vi "lugre.vi"(0 "stribeck velocity":dbl, 1 "bristle stiffness":dbl, 2 "bristle damping":dbl, 3 "viscous friction":dbl, 4 "stiction friction":dbl, 5 "columb friction":dbl, 6 "velocity":dbl, 8 "F before compensation":dbl, 9 "time sampling":dbl, 11 "tracking error":dbl, 13 "observer gain":dbl) -> (14 "F":dbl, 15 "compensated F":dbl)   [LabVIEW 2012]
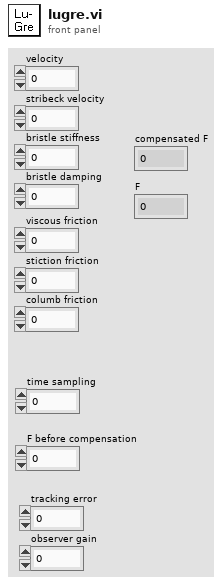
[diagram p1: front panel]
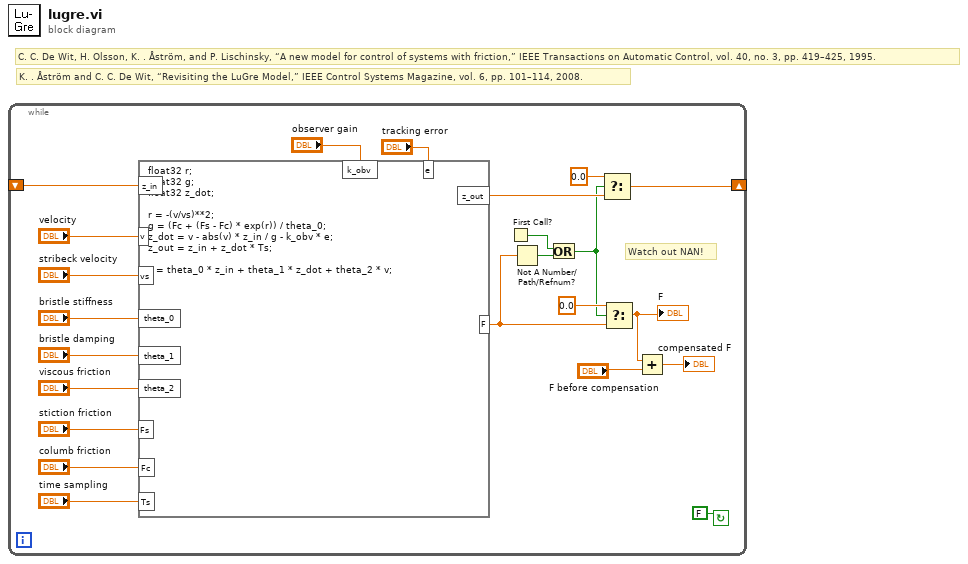
[diagram p0: block diagram]
diagram:
  # "K. . Åström and C. C. De Wit, “Revisiting the LuGre Model,” IEEE Control Systems Magazine, vol. 6, pp. 101–114, 2008."
  # "C. C. De Wit, H. Olsson, K. . Åström, and P. Lischinsky, “A new model for control of systems with friction,” IEEE Transactions on Automatic Control, vol. 40, no. 3, pp. 419–425, 1995."
  n1 = while {
    shift-right: [w4] -> _
    shift-left: _ -> [w14]
    stop <- FALSE continue-if-true
    # "Watch out NAN!"
    n2 = formula code="float32 r;\nfloat32 g;\nfloat32 z_dot;\n\nr = -(v/vs)**2;\ng = (Fc + (Fs - Fc) * exp(r)) / theta_0;\nz_dot = v - abs(v) * z_in / g - k_obv * e;\nz_out = z_in + z_dot * Ts;\n\nF = theta_0 * z_in + theta_1 * z_dot + theta_2 * v;"("v"="velocity", "vs"="stribeck velocity", "theta_0"="bristle stiffness", "theta_1"="bristle damping", "theta_2"="viscous friction", "Fs"="stiction friction", "Fc"="columb friction", "z_in"=w14, "Ts"="time sampling", "k_obv"="observer gain", "e"="tracking error") -> ("z_out"=w13:dbl, "F"=w8:dbl)
    n3 = First Call?() -> (First Call?: T/F=w6:bool)
    n4 = Not A Number/Path/Refnum?(number/path/refnum=w8) -> (NaN/Path/Refnum?=w7:bool)
    n5 = Or(x=w6, y=w7) -> (x .or. y?=w5:bool)
    n6 = Select(t=0.0, s=w5, f=w13) -> (s? t:f=w4:dbl)
    n7 = Select(t=0.0, s=w5, f=w8) -> (s? t:f=w3:dbl)
    "F" <- w3
    n8 = Add(x=w3, y="F before compensation") -> (x+y=→"compensated F":dbl)
  }
